vi "save_images.vi"(4 "ul_ar_pxar_capt_image":u16[][][](array[numeric]), 6 "ul_ar_pxar_orig_pattern":u16[][][](array[numeric]), 10 "p_experiment_path":path, 11 "number of fringes":dbl=4.0) -> ()   [LabVIEW 2011]
uses:
  global_vars.vi
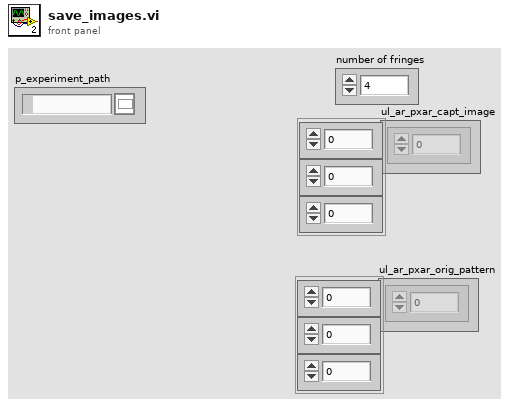
[diagram p1: front panel]
types:
  T1 = typedef "Image Type" = u32
  T2 = typedef "IMAQ Image.ctl" = refnum<image>
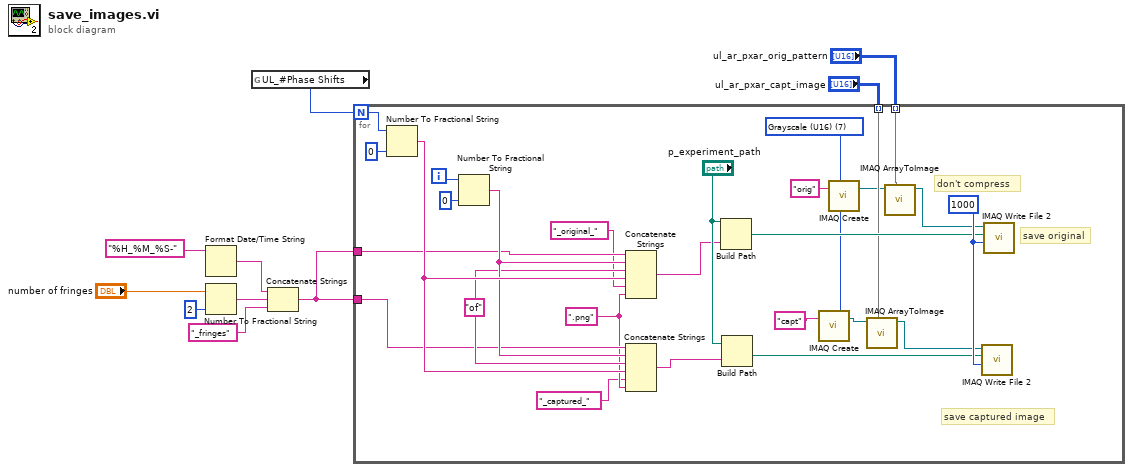
[diagram p0: block diagram]
diagram:
  n1 = Format Date/Time String(time format string (%c)="%H_%M_%S-") -> (date/time string=w9:string)  [unwired: 2 in]
  n2 = Number To Fractional String(number="number of fringes", precision (6)=i16 2) -> (F-format string=w8:string)  [unwired: 2 in]
  n3 = global read "global_vars.vi" "UL_#Phase Shifts"() -> (w4:i32)
  n4 = Concatenate Strings(w9, w8, "_fringes" ("string")) -> (w3:string)
  n5 = for {
    N: w4 -> [w33]
    tunnel: w3 -> [w26]
    tunnel: w3 -> [w23]
    tunnel: "ul_ar_pxar_orig_pattern" -> [w18] mode=indexing
    tunnel: "ul_ar_pxar_capt_image" -> [w19] mode=indexing
    i -> [w29]
    w12 = T1 7 items=["Grayscale (U8)", "Grayscale (I16)", "Grayscale (SGL)", "Complex (CSG)", "RGB (U32)", "HSL (U32)", "RGB (U64)", "Grayscale (U16)"] ("Image Type")
    w22 = ".png" ("string")
    w27 = "of" ("string")
    w37 = u32 1000 ("Image Quality")
    # "don't compress"
    # "save captured image"
    # "save original"
    n6 = Number To Fractional String(number=w33, precision (6)=i16 0) -> (F-format string=w31:string)  [unwired: 2 in]
    n7 = Number To Fractional String(number=w29, precision (6)=i16 0) -> (F-format string=w28:string)  [unwired: 2 in]
    n8 = Concatenate Strings(w26, w28, w27, w31, "_original_" ("name or relative path"), w22) -> (w25:string)
    n9 = Concatenate Strings(w23, w28, w27, w31, "_captured_" ("name or relative path"), w22) -> (w24:string)
    n10 = Build Path(base path="p_experiment_path", name or relative path=w25) -> (appended path=w34:path)
    n11 = Build Path(base path="p_experiment_path", name or relative path=w24) -> (appended path=w35:path)
    n12 = call "IMAQ Create"("Image Name"="capt", "Image Type"=w12) -> ("New Image"=w16:T2)  [unwired: 2 in, 2 out]
    n13 = call "IMAQ Create"("Image Name"="orig", "Image Type"=w12) -> ("New Image"=w11:T2)  [unwired: 2 in, 2 out]
    n14 = call "IMAQ ArrayToImage"("Image Pixels (U16)"=w19, "Image"=w16) -> ("Image Out"=w20:T2)  [unwired: 8 in, 1 out]
    n15 = call "IMAQ ArrayToImage"("Image Pixels (U16)"=w18, "Image"=w11) -> ("Image Out"=w17:T2)  [unwired: 8 in, 1 out]
    n16 = call-poly "IMAQ Write File 2"("Image Quality"=w37, "File Path"=w35, "Image"=w20) -> ()  [unwired: 7 in, 2 out]
    n17 = call-poly "IMAQ Write File 2"("Image Quality"=w37, "File Path"=w34, "Image"=w17) -> ()  [unwired: 7 in, 2 out]
  }
